vi "TempRange_To_DivExp.vi"(10 "Range":string) -> (0 "Exp":string, 2 "Div":dbl)   [LabVIEW 2017]
panel:
  in  "exp":string[](array[string])=["%.;%+0.2f", "%.;%+0.2f", "%.;%+0.2f", "%.;%+0.1f", "%.;%+0.2f", "%.;%+0.2f", "%.;%+0.2f", "%.;%+0.1f"]
  in  "div":dbl[](array[numeric])=[0.005, 0.01, 0.025, 0.1, 0.005, 0.01, 0.025, 0.1]
  in  "RangeCode":string[](array[string])=["100degC", "200degC", "500degC", "2000degC", "150degF", "300degF", "750degF", "3000degF"]
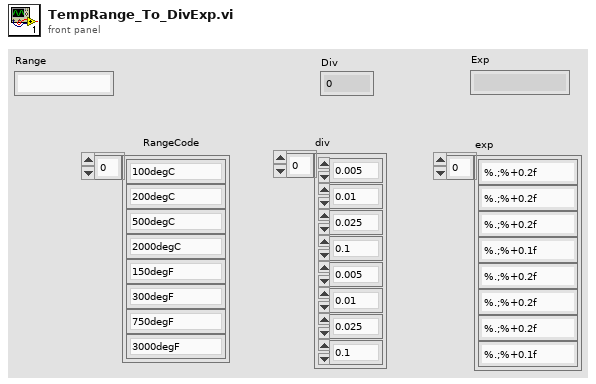
[diagram p1: front panel]
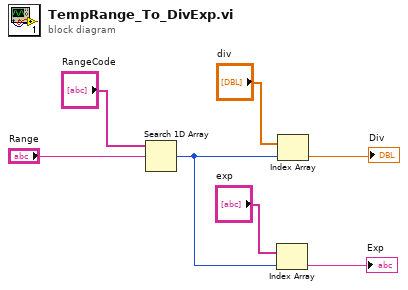
[diagram p0: block diagram]
diagram:
  n1 = Search 1D Array(1D array="RangeCode", element="Range") -> (index of element=w3:i32)  [unwired: 1 in]
  n2 = Index Array(array="exp", index=w3) -> (element=→"Exp":string)
  n3 = Index Array(array="div", index=w3) -> (element=→"Div":dbl)
